vi "Read Address.vi"(8 "error in (no error)":errorcluster, 11 "Simulator in":refnum<class "Simulator.lvclass">) -> (0 "error out":errorcluster, 2 "Address":refnum<visa-resource-name>, 3 "Simulator out":refnum<class "Simulator.lvclass">)   [LabVIEW 2018, in "Simulator.lvclass"]
uses:
  Simulator.lvclass
  Instrument/Instrument.lvclass
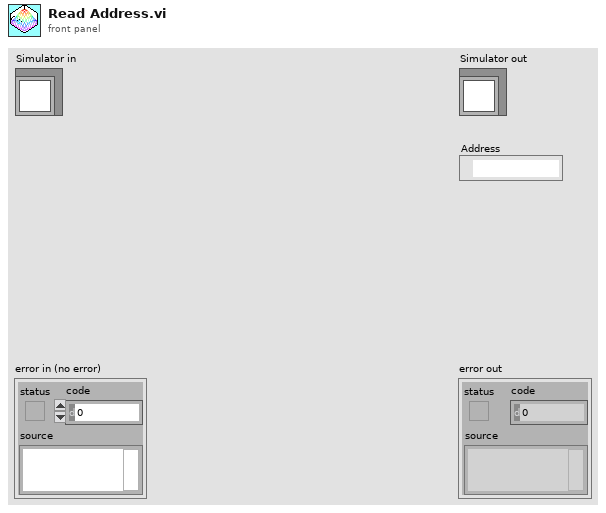
[diagram p1: front panel]
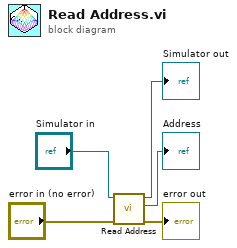
[diagram p0: block diagram]
diagram:
  n1 = call-parent "Read Address.vi"("error in (no error)"="error in (no error)", "Instrument in"="Simulator in") -> ("error out"=→"error out":errorcluster, "Address"=→"Address":refnum<visa-resource-name>, "Instrument out"=→"Simulator out":refnum<class "Simulator.lvclass">)  [unwired: 7 in]
